vi "SetParam.vi"(8 "error in (no error)":errorcluster, 10 "homogeneity_completeness_v_measure":cluster{"beta":dbl, "Returns":string}={"beta"=1.0, "Returns"="homogeneity"}, 11 "Homogeneity_C_V_M.lvclass":refnum<class "Homogeneity_C_V_M.lvclass">) -> (0 "error out":errorcluster, 3 "Homogeneity_C_V_M.lvclass":refnum<class "Homogeneity_C_V_M.lvclass">)   [LabVIEW 2020, in "Homogeneity_C_V_M.lvclass"]
doc: "Set parameters"
uses:
  Homogeneity_C_V_M.lvclass
  Homogeneity_C_V_M.lvclass/Homogeneity_C_V_M.ctl
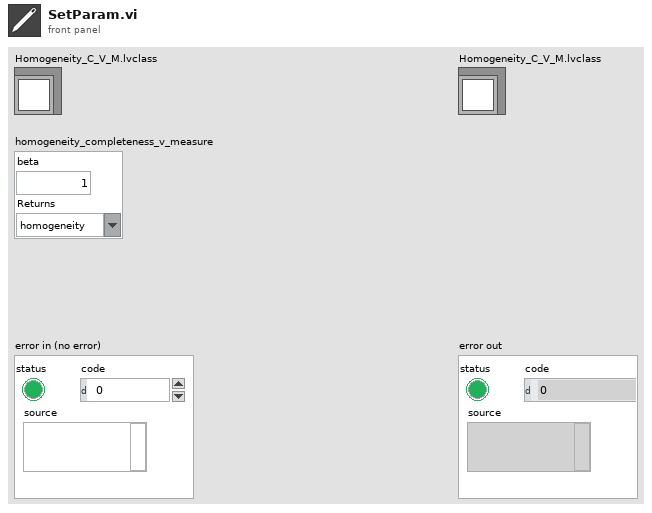
[diagram p1: front panel]
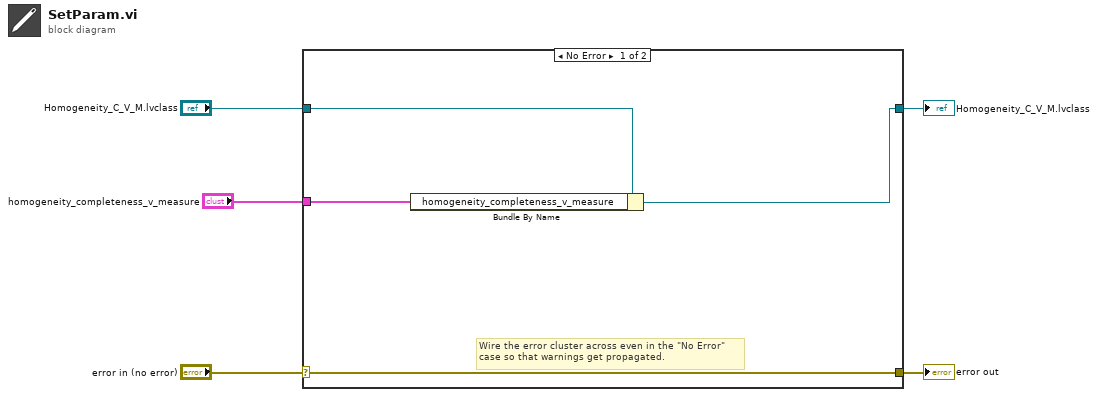
[diagram p0: block diagram]
diagram:
  n1 = case shown="No Error" "error in (no error)" {
    selector: "error in (no error)" -> [w9 w11]
    tunnel: [w9 w11] -> w4
    tunnel: [w6 w10] -> w2
    tunnel: "Homogeneity_C_V_M.lvclass" -> [w8 w10]
    tunnel: "homogeneity_completeness_v_measure" -> [w7 _]
    frame No Error {
      # "Wire the error cluster across even in the \"No Error\"\ncase so that warnings get propagated."
      n2 = Bundle By Name(cluster=w8, "homogeneity_completeness_v_measure"=w7) -> (w6:refnum<class "Homogeneity_C_V_M.lvclass">)
    }
    frame Error {
    }
  }
  "error out" <- w4
  "Homogeneity_C_V_M.lvclass" <- w2
